vi "LEP_RV_LoadBuildConfig.vi"(0 "error in (no error)":errorcluster) -> (1 "Status":T1(ring)=enum."EmptyTopLevelVIPath", 2 "Config":T2={"Enable debugging"=FALSE, "Debug Options"=0, "Use stack variables"=FALSE, "Generate serial only"=FALSE, "Generate guard code"=TRUE, "Generate Integer Only"=TRUE, "Generate C Function Calls"=TRUE, "ExpressionFolding"=FALSE, "Constant Allocation"=0, "Constant Deallocation"=0, "Build Specification ID"="", "Preprocessor symbols (define)"="", "Compiler Flags"="", "Linker Flags"="", "Mode"=1, "Optimization"=2, "Optimize for time"=FALSE, "Enable cross-module optimization"=FALSE, "Include paths"=[], "Optimize heap size"=FALSE, "Use MicroLib"=FALSE, "Debug Mode"=2, "Enable profile information"=FALSE, "Host name"="", "Use DHCP"=TRUE, "IP address"="0.0.0.0", "Subnet mask"="", "Gateway"="0.0.0.0", "Primary DNS"="0.0.0.0", "Secondary DNS"="0.0.0.0", "MAC in target memory"=TRUE, "MAC address"="", "Console output"=0, "Target serial port"=1} {"Constant Deallocation" items=["Out of Scope", "VI End", "Application End"]; "Constant Allocation" items=["First Use", "Containing Loop", "VI Initialization", "Application Initialization"]; "Target serial port" items=["0", "1", "2", "3"]; "Console output" items=["Processor status window", "Serial port"]; "Optimization" items=["Level 0 (-O0)", "Level 1 (-O1)", "Level 2 (-O2)", "Level 3 (-O3)"]; "Mode" items=["ARM-Mode", "Thumb-Mode"]; "Debug Options" items=["Use ULINK Debugger", "Use Simulator"]; "Debug Mode" items=["Instrumented (serial port)", "Instrumented (TCP/IP)", "Non-instrumented (JTAG/USB)"]}, 3 "error out":errorcluster)   [LabVIEW 2011]
doc: "Populates <B>Config</B> with the embedded project settings of the current project."
uses:
  LEP_RV_Config.ctl
  <vilib>/Platform/EmbProject/Plugins/utilities/LEP_Utilities_GetSetProjectData_Variant.vi
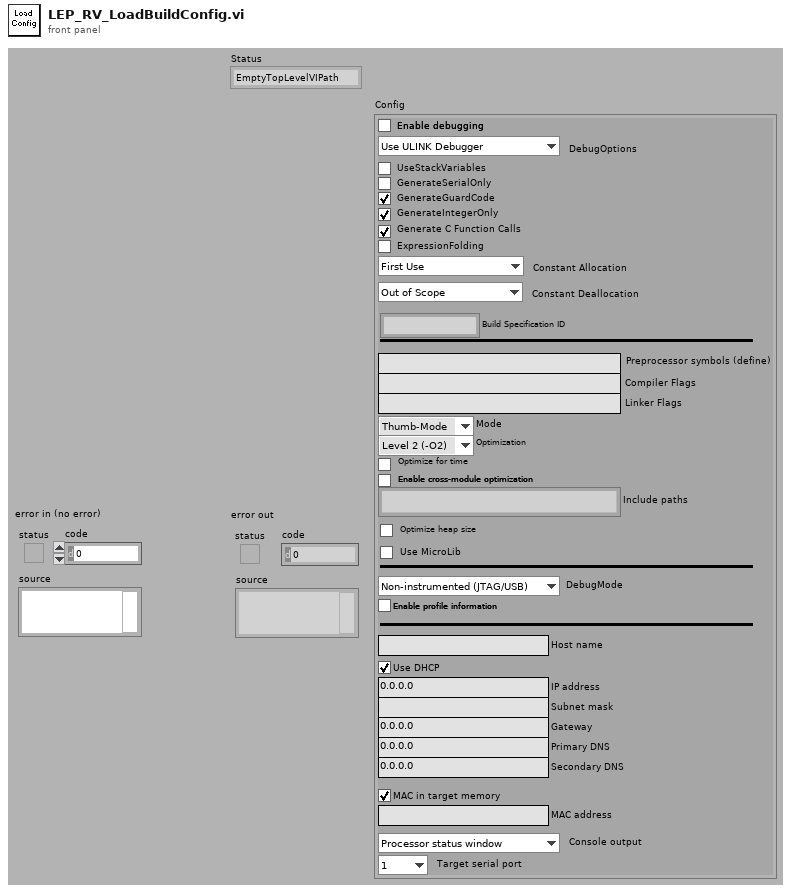
[diagram p1: front panel]
types:
  T1 = enum16{"NoErr", "TopLevelVIErr", "EmptyTopLevelVIPath", "CGenErr", "CpySuppFilesErr", "ProjectInfoErr", "NoTopLevelVIErr", "CreateBuildFolderErr", "EmptyBuildFolderErr", "LoadConfigErr", "BildToolsErr", "CompileErr", "LinkError", "DebugInfoErr", "NotFoundErr", "AccessErr", "ExecErr", "UnknownErr"}
  T2 = typedef "LEP_RV_Config.ctl" = cluster{"Enable debugging":bool, "Debug Options":u16, "Use stack variables":bool, "Generate serial only":bool, "Generate guard code":bool, "Generate Integer Only":bool, "Generate C Function Calls":bool, "ExpressionFolding":bool, "Constant Allocation":u16, "Constant Deallocation":u16, "Build Specification ID":string, "Preprocessor symbols (define)":string, "Compiler Flags":string, "Linker Flags":string, "Mode":u16, "Optimization":u16, "Optimize for time":bool, "Enable cross-module optimization":bool, "Include paths":path[], "Optimize heap size":bool, "Use MicroLib":bool, "Debug Mode":u16, "Enable profile information":bool, "Host name":string, "Use DHCP":bool, "IP address":string, "Subnet mask":string, "Gateway":string, "Primary DNS":string, "Secondary DNS":string, "MAC in target memory":bool, "MAC address":string, "Console output":u16, "Target serial port":u16}
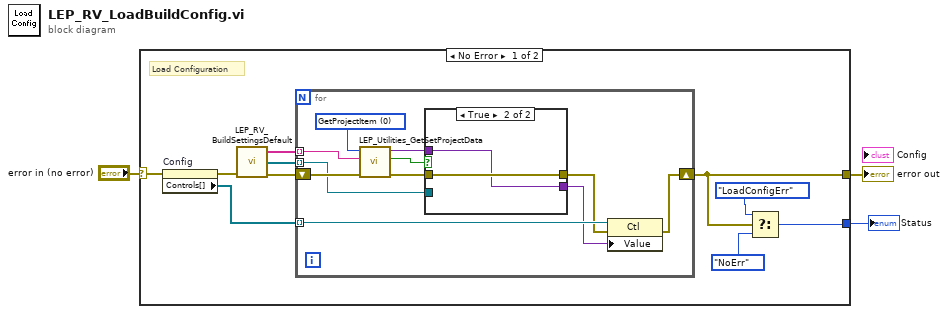
[diagram p0: block diagram]
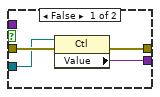
[diagram p2: hidden frame]
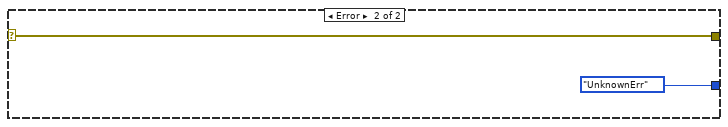
[diagram p3: hidden frame]
diagram:
  n1 = case shown="No Error" "error in (no error)" {
    selector: "error in (no error)" -> [w10 w32]
    tunnel: [w7 w32] -> w2
    tunnel: [w6 T1."UnknownErr" ("Errors")] -> w1
    frame No Error {
      # "Load Configuration"
      n2 = property on="Config" class="Clust (strict)"(error in=w10) -> (error out=w9:errorcluster, "Controls[]"=w8:refnum<vi>[])  [unwired: 1 in, 1 out]
      n3 = call "LEP_RV_BuildSettingsDefault.vi"("error in (no error)"=w9) -> ("error out"=w13:errorcluster, "Default Values"=w12:refnum<vi>[], "Attribute Name"=w11:string[])  [unwired: 2 in]
      n4 = for {
        shift-right: [w17] -> w7
        shift-left: w13 -> [w24]
        tunnel: w12 -> [w15] mode=indexing
        tunnel: w11 -> [w23] mode=indexing
        tunnel: w8 -> [w18] mode=indexing
        w22 = u16 0 items=["GetProjectItem", "SetProjectItem"] ("Command")
        n5 = call-poly <vilib>:"LEP_Utilities_GetSetProjectData.vi"("error in"=w24, "ItemName"=w23, "Command"=w22) -> ("error out"=w19:errorcluster, "Found/Replaced?"=w21:bool, "Variant Out"=w20:variant)  [unwired: 6 in]
        n6 = case shown="True" w21 {
          tunnel: w20 -> [_ w29]
          tunnel: w19 -> [w28 w30]
          tunnel: [w27 w30] -> w16
          tunnel: w15 -> [w26 _]
          tunnel: [w25 w29] -> w14
          frame False {
            n7 = property class="Ctl"(reference=w26, error in=w28) -> (error out=w27:errorcluster, "Value"=w25:variant)  [unwired: 1 out]
          }
          frame True {
          }
        }
        n8 = property class="Ctl"(reference=w18, error in=w16, "Value"=w14) -> (error out=w17:errorcluster)  [unwired: 1 out]
      }
      n9 = Select(t=T1."LoadConfigErr" ("Errors"), s=w7, f=T1."NoErr" ("Errors")) -> (s? t:f=w6:T1)
    }
    frame Error {
    }
  }
  "error out" <- w2
  "Status" <- w1
